vi "Multi Axis Waveform Acquisition.vi"() -> ()   [LabVIEW 2012]
uses:
  <vilib>/Utility/file.llb/Read From Spreadsheet File (DBL).vi
  <vilib>/Utility/file.llb/Write To Spreadsheet File (DBL).vi
  Madlib.dll
panel:
  in  "Ramp Z from (um)":dbl format="%.4f"
  in  "Ramp Z to (um)":dbl=1.0 format="%.4f"
  in  "Ramp Y from (um)":dbl format="%.4f"
  in  "Ramp Y to (um)":dbl=1.0 format="%.4f"
  in  "Ramp X to (um)":dbl=1.0 format="%.4f"
  out "Z Graph":dbl[](graph)
  out "Y Graph":dbl[](graph)
  in  "Ramp X from (um)":dbl format="%.4f"
  in  "iterations":u16=1
  in  "Datapoints Per Axis":i32=100
  in  "Load Z Waveform From":path
  in  "Load Y Waveform From":path
  in  "Rate (ms)":dbl=1.0 format="%.4f"
  in  "Write Waveform To (optional)":path
  in  "Load X Waveform From":path
  out "X Graph":dbl[](graph)
  # "Multi Axis Waveform Acquisition"
  # "This example demonstrates the two step process of triggering a waveform read/write on multiple axes. Position control data (separated by spaces) is loaded from specified basic text files (Load Waveform From) and position data read from the axes is appended to a file (Write Waveform To)."
  # "Step 1"
  # "Step 2"
  # "Step 3 --"
  # "Specify the rate of commands/reads, the number of datapoints per iteration, and the number of iterations. Optional: Specify a file  below to save ADC data from the scan."
  # "Load command waveforms for each axis from a file or leave the field/s blank to generate a ramp based on the available controls."
  # "Run the vi. The graphs below will show the ADC data returned from the MCL_WfmaTriggerAndRead() function."
  # "X axis"
  # "Y axis"
  # "Z axis"
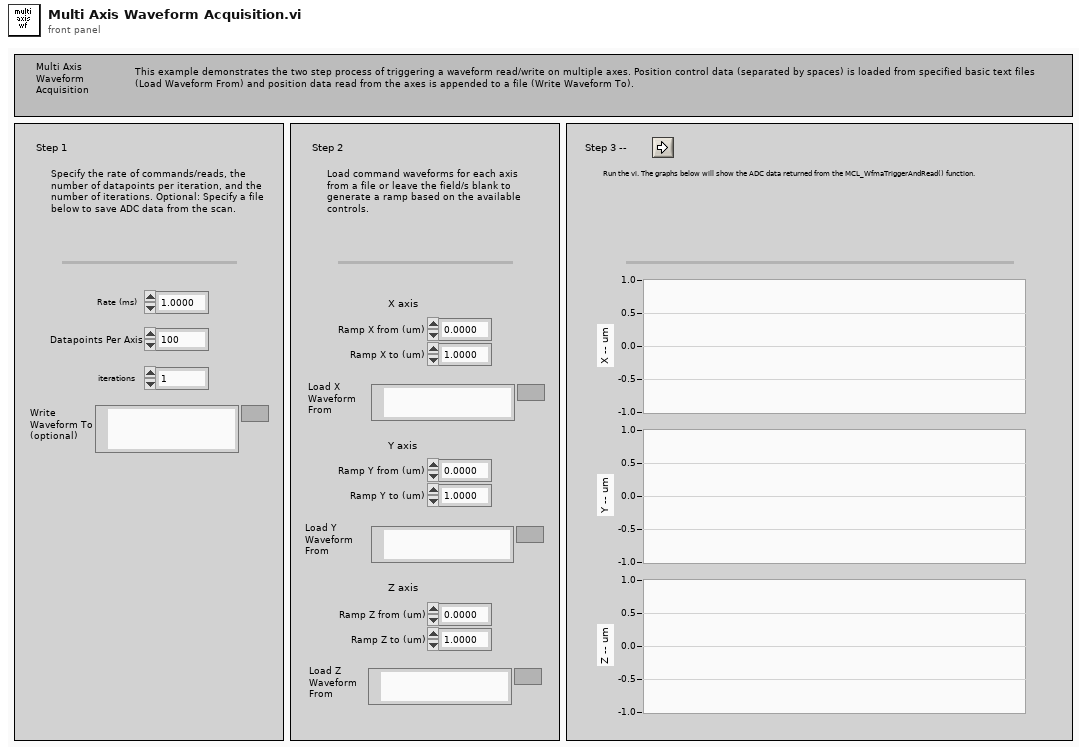
[diagram p1: front panel]
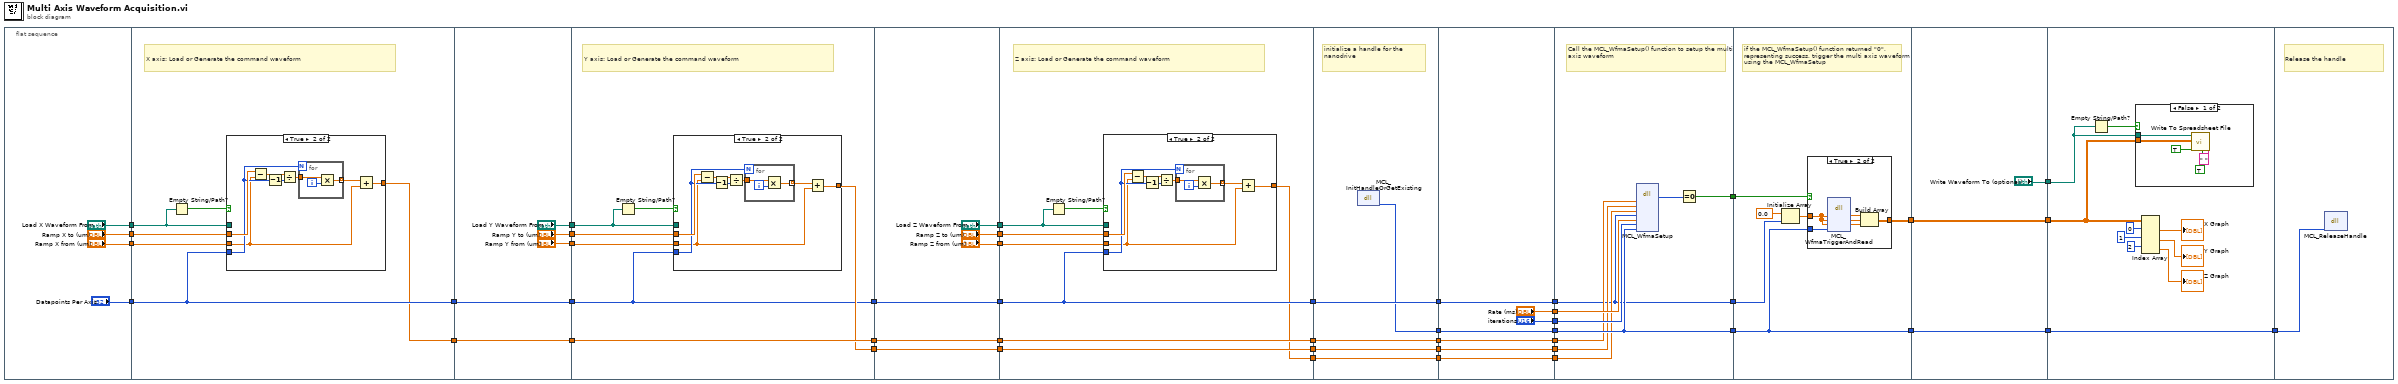
[diagram p0: block diagram]
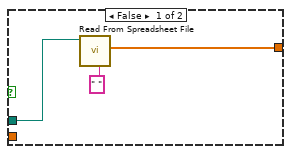
[diagram p2: hidden frame]
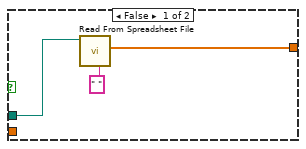
[diagram p3: hidden frame]
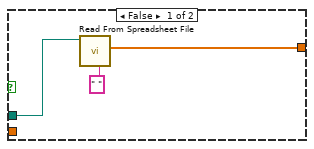
[diagram p4: hidden frame]
diagram:
  n1 = flat-sequence {
    tunnel: ["Load X Waveform From"] -> w43
    tunnel: ["Ramp X from (um)"] -> w37
    tunnel: ["Ramp X to (um)"] -> w36
    tunnel: ["Datapoints Per Axis"] -> w33
    tunnel: w43 -> [w52]
    tunnel: w37 -> [w55]
    tunnel: w36 -> [w54]
    tunnel: [w51] -> w35
    tunnel: [w53] -> w34
    tunnel: w33 -> [w53]
    tunnel: w35 -> [w72]
    tunnel: w34 -> [w73]
    tunnel: ["Load Y Waveform From"] -> w32
    tunnel: ["Ramp Y to (um)"] -> w31
    tunnel: ["Ramp Y from (um)"] -> w30
    tunnel: [w73] -> w29
    tunnel: [w72] -> w28
    tunnel: w32 -> [w81]
    tunnel: w31 -> [w80]
    tunnel: w30 -> [w79]
    tunnel: w29 -> [w76]
    tunnel: [w78] -> w27
    tunnel: w28 -> [w78]
    tunnel: [w77] -> w26
    tunnel: [w76] -> w25
    tunnel: w27 -> [w101]
    tunnel: [w101] -> w24
    tunnel: w26 -> [w100]
    tunnel: [w100] -> w22
    tunnel: [w99] -> w20
    tunnel: w25 -> [w99]
    tunnel: ["Load Z Waveform From"] -> w18
    tunnel: ["Ramp Z to (um)"] -> w17
    tunnel: ["Ramp Z from (um)"] -> w16
    tunnel: w24 -> [w109]
    tunnel: [w109] -> w23
    tunnel: w22 -> [w108]
    tunnel: [w108] -> w21
    tunnel: w20 -> [w104]
    tunnel: [w104] -> w19
    tunnel: w18 -> [w105]
    tunnel: w17 -> [w107]
    tunnel: w16 -> [w106]
    tunnel: [w103] -> w15
    tunnel: [w124] -> w41
    tunnel: w23 -> [w127]
    tunnel: w21 -> [w126]
    tunnel: w19 -> [w128]
    tunnel: w15 -> [w125]
    tunnel: [w128] -> w13
    tunnel: [w127] -> w11
    tunnel: [w126] -> w9
    tunnel: [w125] -> w7
    tunnel: w41 -> [w135]
    tunnel: [w135] -> w40
    tunnel: ["iterations"] -> w39
    tunnel: ["Rate (ms)"] -> w38
    tunnel: [w132] -> w14
    tunnel: w13 -> [w132]
    tunnel: [w131] -> w12
    tunnel: w11 -> [w131]
    tunnel: [w130] -> w10
    tunnel: w9 -> [w130]
    tunnel: [w129] -> w8
    tunnel: w7 -> [w129]
    tunnel: [w144] -> w45
    tunnel: w40 -> [w142]
    tunnel: [w142] -> w44
    tunnel: w39 -> [w140]
    tunnel: w38 -> [w141]
    tunnel: w14 -> [w136]
    tunnel: w12 -> [w139]
    tunnel: w10 -> [w138]
    tunnel: w8 -> [w137]
    tunnel: [w136] -> w3
    tunnel: w45 -> [w148]
    tunnel: w44 -> [w146]
    tunnel: [w146] -> w6
    tunnel: w3 -> [w147]
    tunnel: [w145] -> w2
    tunnel: w6 -> [w159]
    tunnel: [w159] -> w5
    tunnel: ["Write Waveform To (optional)"] -> w4
    tunnel: w2 -> [w157]
    tunnel: [w157] -> w1
    tunnel: [w169] -> w42
    tunnel: w5 -> [w169]
    tunnel: w4 -> [w160]
    tunnel: w1 -> [w162]
    tunnel: w42 -> [w175]
    frame #0 {
    }
    frame #1 {
      # "X axis: Load or Generate the command waveform"
      n2 = Empty String/Path?(string/path=w52) -> (empty?=w50:bool)
      n3 = case shown="True" w50 {
        tunnel: w52 -> [w58 _]
        tunnel: w55 -> [_ w59]
        tunnel: w54 -> [_ w66]
        tunnel: [w56 w60] -> w51
        tunnel: w53 -> [_ w63]
        frame False {
          n4 = call-poly <vilib>:"Read From Spreadsheet File.vi"("delimiter (\\t)"=" ", "file path (dialog if empty)"=w58) -> ("first row"=w56:dbl[])  [unwired: 3 in, 6 out]
        }
        frame True {
          n5 = Subtract(x=w66, y=w59) -> (x-y=w65:dbl)
          n6 = Decrement(x=w63) -> (x-1=w62:i32)
          n7 = Divide(x=w65, y=w62) -> (x/y=w64:dbl)
          n8 = for {
            N: w63 -> [_]
            tunnel: w64 -> [w68]
            tunnel: [w67] -> w61 mode=indexing
            i -> [w69]
            n9 = Multiply(x=w68, y=w69) -> (x*y=w67:dbl)
          }
          n10 = Add(x=w61, y=w59) -> (x+y=w60:dbl[])
        }
      }
    }
    frame #2 {
    }
    frame #3 {
      # "Y axis: Load or Generate the command waveform"
      n11 = Empty String/Path?(string/path=w81) -> (empty?=w75:bool)
      n12 = case shown="True" w75 {
        tunnel: w81 -> [w84 _]
        tunnel: w79 -> [_ w85]
        tunnel: w80 -> [_ w92]
        tunnel: [w82 w86] -> w77
        tunnel: w76 -> [_ w89]
        frame False {
          n13 = call-poly <vilib>:"Read From Spreadsheet File.vi"("delimiter (\\t)"=" ", "file path (dialog if empty)"=w84) -> ("first row"=w82:dbl[])  [unwired: 3 in, 6 out]
        }
        frame True {
          n14 = Subtract(x=w92, y=w85) -> (x-y=w91:dbl)
          n15 = Decrement(x=w89) -> (x-1=w88:i32)
          n16 = Divide(x=w91, y=w88) -> (x/y=w90:dbl)
          n17 = for {
            N: w89 -> [_]
            tunnel: w90 -> [w94]
            tunnel: [w93] -> w87 mode=indexing
            i -> [w95]
            n18 = Multiply(x=w94, y=w95) -> (x*y=w93:dbl)
          }
          n19 = Add(x=w87, y=w85) -> (x+y=w86:dbl[])
        }
      }
    }
    frame #4 {
    }
    frame #5 {
      # "Z axis: Load or Generate the command waveform"
      n20 = Empty String/Path?(string/path=w105) -> (empty?=w102:bool)
      n21 = case shown="True" w102 {
        tunnel: w105 -> [w112 _]
        tunnel: w106 -> [_ w114]
        tunnel: w107 -> [_ w120]
        tunnel: [w110 w113] -> w103
        tunnel: w104 -> [_ w117]
        frame False {
          n22 = call-poly <vilib>:"Read From Spreadsheet File.vi"("delimiter (\\t)"=" ", "file path (dialog if empty)"=w112) -> ("first row"=w110:dbl[])  [unwired: 3 in, 6 out]
        }
        frame True {
          n23 = Subtract(x=w120, y=w114) -> (x-y=w119:dbl)
          n24 = Decrement(x=w117) -> (x-1=w116:i32)
          n25 = Divide(x=w119, y=w116) -> (x/y=w118:dbl)
          n26 = for {
            N: w117 -> [_]
            tunnel: w118 -> [w122]
            tunnel: [w121] -> w115 mode=indexing
            i -> [w123]
            n27 = Multiply(x=w122, y=w123) -> (x*y=w121:dbl)
          }
          n28 = Add(x=w115, y=w114) -> (x+y=w113:dbl[])
        }
      }
    }
    frame #6 {
      # "initialize a handle for the nanodrive"
      n29 = dll-call lib="C:/Users/Labview/Desktop/SRR/Madlib_x64/Labview Examples/MADLib.dll" fn="MCL_InitHandleOrGetExisting" label="InitHandle"() -> ("handle"=w124:i32)  [unwired: 3 in, 2 out]
    }
    frame #7 {
    }
    frame #8 {
      # "Call the MCL_WfmaSetup() function to setup the multi axis waveform"
      n30 = dll-call lib="C:/Users/Labview/Desktop/SRR/Madlib_x64/Labview Examples/Madlib.dll" fn="MCL_WfmaSetup" label="WfmaSetup"("wfDacX"=w139, "wfDacY"=w138, "wfDacZ"=w137, "dataPointsPerAxis"=w136, "milliseconds"=w141, "iterations"=w140, "handle"=w142) -> ("error code"=w143:i32)  [unwired: 10 in, 2 out]
      n31 = Equal To 0?(x=w143) -> (x = 0?=w144:bool)
    }
    frame #9 {
      # "if the MCL_WfmaSetup() function returned \"0\", representing success, trigger the multi axis waveform using the MCL_WfmaSetup"
      n32 = Initialize Array(0.0, w147) -> (w150:dbl[])
      n33 = case shown="True" w148 {
        tunnel: w150 -> [_ w155]
        tunnel: w146 -> [_ w156]
        tunnel: [_ w151] -> w145
        frame False {
        }
        frame True {
          n34 = dll-call lib="C:/Users/Labview/Desktop/SRR/Madlib_x64/Labview Examples/MADLib.dll" fn="MCL_WfmaTriggerAndRead" label="WfmaSetup"("wfAdcX"=w155, "wfAdcY"=w155, "wfAdcZ"=w155, "handle"=w156) -> ("wfAdcX"=w154:dbl[], "wfAdcY"=w153:dbl[], "wfAdcZ"=w152:dbl[])  [unwired: 4 in, 3 out]
          n35 = Build Array(w154, w153, w152) -> (w151:dbl[][])
        }
      }
    }
    frame #10 {
    }
    frame #11 {
      n36 = Empty String/Path?(string/path=w160) -> (empty?=w161:bool)
      n37 = case shown="False" w161 {
        tunnel: w162 -> [w173 _]
        tunnel: w160 -> [w170 _]
        frame False {
          n38 = call-poly <vilib>:"Write To Spreadsheet File.vi"("delimiter (\\t)"=" ", "transpose? (no:F)"=TRUE, "append to file? (new file:F)"=TRUE, "2D data"=w173, "file path (dialog if empty)"=w170) -> ()  [unwired: 2 in, 2 out]
        }
        frame True {
        }
      }
      n39 = Index Array(array=w162, index (row) #1=0 ("index (row)"), index (row) #2=1 ("index (row)"), index (row) #3=2 ("index (row)")) -> (element #1=→"X Graph":dbl[], element #2=→"Y Graph":dbl[], element #3=→"Z Graph":dbl[])  [unwired: 3 in]
    }
    frame #12 {
      # "Release the handle"
      n40 = dll-call lib="C:/Users/Labview/Desktop/SRR/Madlib_x64/Labview Examples/MADLib.dll" fn="MCL_ReleaseHandle"("handle"=w175) -> ()  [unwired: 4 in, 3 out]
    }
  }
